vi "AlazarDSPGetModules.vi"(0 "Handle":u64, 1 "error in (no error)":errorcluster) -> (2 "Handle":u64, 3 "Return Code":u32, 4 "DSP Modules":u64[](array[numeric]), 5 "error out":errorcluster)   [LabVIEW 2018]
uses:
  ATSApi.dll
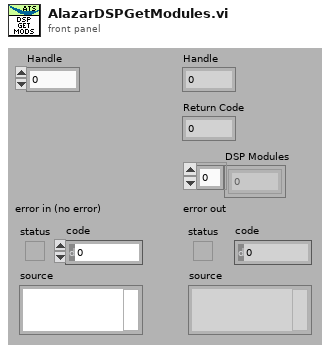
[diagram p1: front panel]
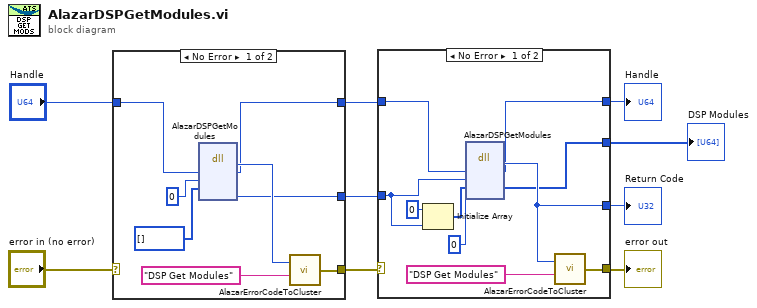
[diagram p0: block diagram]
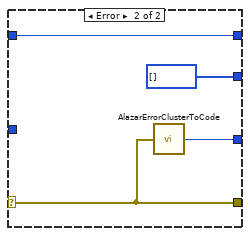
[diagram p2: hidden frame]
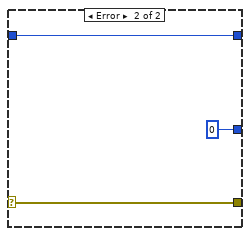
[diagram p3: hidden frame]
diagram:
  n1 = case shown="No Error" "error in (no error)" {
    selector: "error in (no error)" -> [_ w20]
    tunnel: [w14 w20] -> w1
    tunnel: "Handle" -> [w17 w19]
    tunnel: [w13 w19] -> w6
    tunnel: [w11 0] -> w7
    frame No Error {
      n2 = dll-call lib="ATSApi.dll" fn="AlazarDSPGetModules"("handle"=w17, "numEntries"=u32 0, "modules"=u64[] []) -> ("return type"=w16:u32, "handle"=w13:u64, "numModules"=w11:u32)  [unwired: 6 in, 2 out]
      n3 = call "AlazarErrorCodeToCluster.vi"("Message"="DSP Get Modules", "Error Code"=w16) -> ("error out"=w14:errorcluster)
    }
    frame Error {
    }
  }
  n4 = case shown="No Error" w1 {
    selector: w1 -> [_ w34]
    tunnel: [w27 w34] -> w4
    tunnel: [w29 w33] -> w5
    tunnel: w6 -> [w30 w32]
    tunnel: [w26 w32] -> w3
    tunnel: w7 -> [w25 _]
    tunnel: [w22 u32[] []] -> w2
    frame No Error {
      n5 = Initialize Array(u64 0, w25) -> (w23:u64[])
      n6 = dll-call lib="ATSApi.dll" fn="AlazarDSPGetModules"("handle"=w30, "numEntries"=w25, "modules"=w23, "numModules"=u32 0) -> ("return type"=w29:u32, "handle"=w26:u64, "modules"=w22:u64[])  [unwired: 5 in, 2 out]
      n7 = call "AlazarErrorCodeToCluster.vi"("Message"="DSP Get Modules", "Error Code"=w29) -> ("error out"=w27:errorcluster)
    }
    frame Error {
      n8 = call "AlazarErrorClusterToCode.vi"("error in (no error)"=w34) -> ("Error Code"=w33:u32)
    }
  }
  "Handle" <- w3
  "error out" <- w4
  "Return Code" <- w5
  "DSP Modules" <- w2
